vi "Write Max messagee size to send (octets).vi"(8 "error in (no error)":errorcluster, 10 "Max Messagre Size (octets)":u8, 11 "RawSocket Handler in":refnum<class "RawSocket Handler.lvclass">) -> (0 "error out":errorcluster, 3 "RawSocket Handler out":refnum<class "RawSocket Handler.lvclass">)   [LabVIEW 2020, in "wamplv.lvlib" / "RawSocket Handler.lvclass"]
uses:
  RawSocket Handler.lvclass
  RawSocket Handler.lvclass/RawSocket Handler.ctl
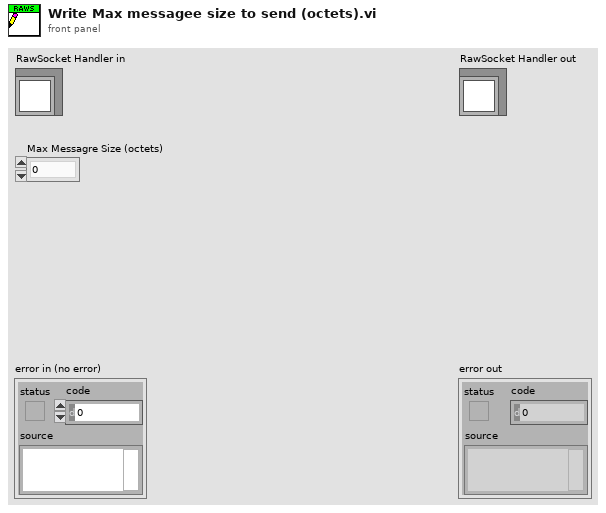
[diagram p1: front panel]
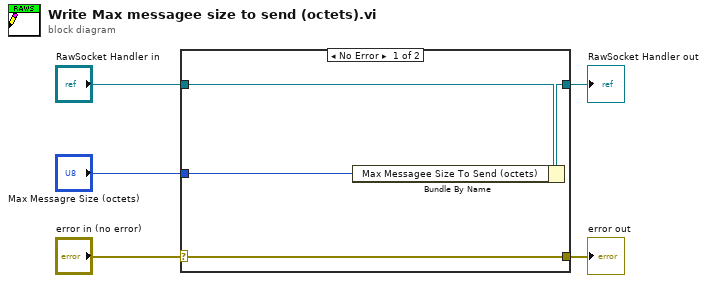
[diagram p0: block diagram]
diagram:
  n1 = case shown="No Error" "error in (no error)" {
    selector: "error in (no error)" -> [w9 w10]
    tunnel: [w9 w10] -> w4
    tunnel: [w7 w11] -> w2
    tunnel: "RawSocket Handler in" -> [w8 w11]
    tunnel: "Max Messagre Size (octets)" -> [w6 _]
    frame No Error {
      n2 = Bundle By Name(cluster=w8, "Max Messagee Size To Send (octets)"=w6) -> (w7:refnum<class "RawSocket Handler.lvclass">)
    }
    frame Error {
    }
  }
  "error out" <- w4
  "RawSocket Handler out" <- w2
